vi "Initialize-status-notifs.vi"(8 "error in (no error)":errorcluster, 11 "Object ref in":T1) -> (0 "error out":errorcluster, 3 "Object ref out":T1)   [LabVIEW 2013, in "SLMControl.lvlib" / "SC-Main.lvclass"]
uses:
  SC-Main.lvclass
  Object-reference.ctl
  SC-Main.lvclass/SC-Main.ctl
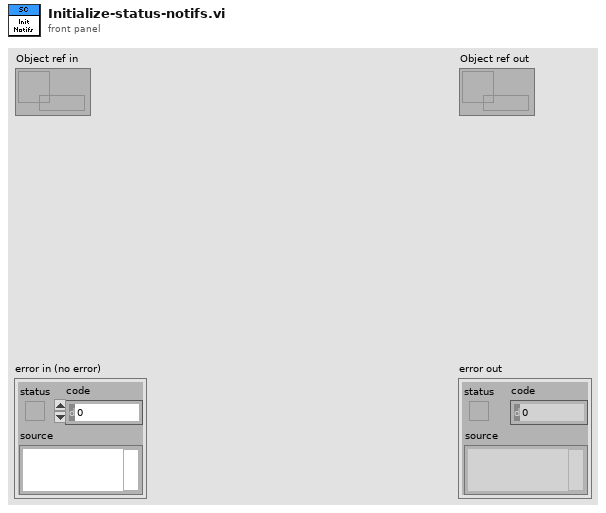
[diagram p1: front panel]
types:
  T1 = typedef "SLMControl.lvlib/SC-Main.lvclass/Object-reference.ctl" = refnum<data-value>
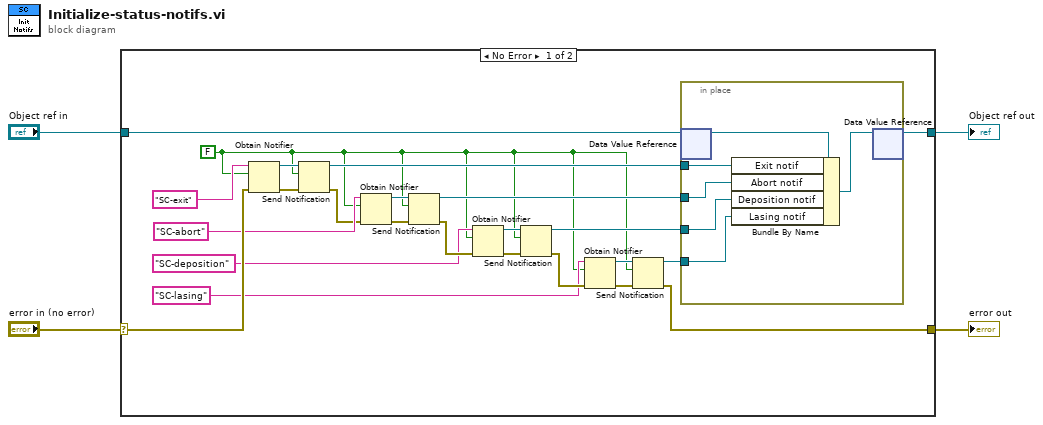
[diagram p0: block diagram]
diagram:
  n1 = case shown="No Error" "error in (no error)" {
    selector: "error in (no error)" -> [w25 w36]
    tunnel: [w12 w36] -> w3
    tunnel: [w27 w35] -> w1
    tunnel: "Object ref in" -> [w28 w35]
    frame No Error {
      w5 = FALSE
      n2 = Obtain Notifier(name (unnamed)="SC-exit", notification data type=w5, error in (no error)=w25) -> (notifier out=w26:refnum<notifier>, error out=w20:errorcluster)  [unwired: 1 in, 1 out]
      n3 = Send Notification(notification=w5, notifier=w26, error in (no error)=w20) -> (notifier out=w21:refnum<notifier>, error out=w17:errorcluster)
      n4 = Obtain Notifier(name (unnamed)="SC-abort", notification data type=w5, error in (no error)=w17) -> (notifier out=w24:refnum<notifier>, error out=w18:errorcluster)  [unwired: 1 in, 1 out]
      n5 = Send Notification(notification=w5, notifier=w24, error in (no error)=w18) -> (notifier out=w19:refnum<notifier>, error out=w14:errorcluster)
      n6 = Obtain Notifier(name (unnamed)="SC-deposition", notification data type=w5, error in (no error)=w14) -> (notifier out=w9:refnum<notifier>, error out=w16:errorcluster)  [unwired: 1 in, 1 out]
      n7 = Send Notification(notification=w5, notifier=w9, error in (no error)=w16) -> (notifier out=w7:refnum<notifier>, error out=w13:errorcluster)
      n8 = Obtain Notifier(name (unnamed)="SC-lasing", notification data type=w5, error in (no error)=w13) -> (notifier out=w8:refnum<notifier>, error out=w15:errorcluster)  [unwired: 1 in, 1 out]
      n9 = Send Notification(notification=w5, notifier=w8, error in (no error)=w15) -> (notifier out=w6:refnum<notifier>, error out=w12:errorcluster)
      n10 = in-place {
        in-place-border: w21 -> [w32]
        in-place-border: w19 -> [w31]
        in-place-border: w7 -> [w30]
        in-place-border: w6 -> [w29]
        n11 = in-place-dvr #1(w28) -> (w34:refnum<class "SC-Main.lvclass">)  [unwired: 1 out]
        n12 = Bundle By Name(cluster=w34, "Exit notif"=w32, "Abort notif"=w31, "Deposition notif"=w30, "Lasing notif"=w29) -> (w33:refnum<class "SC-Main.lvclass">)
        n13 = in-place-dvr #1(w33) -> (w27:T1)  [unwired: 1 out]
      }
    }
    frame Error {
    }
  }
  "error out" <- w3
  "Object ref out" <- w1
